vi "Configuration.vi"() -> ()   [LabVIEW 2021]
uses:
  <vilib>/Analysis/Matrix/Datatypes/RealMatrix.ctl
  Sub VIs/Configuration/Configuration.ctl
  <vilib>/Analysis/Matrix/NI_Matrix.lvlib
panel:
  out "values loded in xml files":T1
  in  "file path (trajectorymat)":path=path "c:/ni-rt/startup/new_trajectoryfile.csv"
  in  "file path (matrixmat)":path=path "c:/ni-rt/startup/matrixmat_default.csv"
  in  "Configuration":T2={"Accelerometer Bias"={"X (m/s)"=0.0, "Y (m/s)"=0.5797, "Z (m/s)"=0.0}, "Gyroscope Bias"={"X (m/s)"=0.0, "Y (m/s)"=0.0, "Z (m/s)"=0.0}, "Steering Motor Gear Ratio"=111.0, "Steering Pully Gear Ratio"=1.0, "Steering Encoder CPR"=500.0, "Steering Motor Max RPM"=4000.0, "Wheelbase (m)"=1.12, "Fork Angle (rad)"=1.3, "Balancing Controller"={"Kp (/s)"=1.3, "Kd (1)"=3.0}, "Max Allowed Steering Angle (rad)"=0.7, "Task Periods"={"Emergency Stop (us)"=10000, "IMU (us)"=10000, "Steering Motor Encoder (us)"=10000, "State Estimator (us)"=10000, "Balancing Controller (us)"=10000, "GNSS (us)"=10000, "Logging (us)"=10000, "Drive Motor (us)"=100000, "Visualization (us)"=100000}, "Drive Motor Gear Ratio"=250.0, "lr"=0.4964, "lf"=0.5986, "lambda"=1.2217, "k1"=0.004472, "k2"=0.09678, "e1_max"=11.331, "Ad_tmin"=0.95971, "Bd_tmin"=0.01, "C_tmin"=2.20588, "D_tmin"=0.0, "Wheel radius"=0.311, "Ad_tmax"=0.95971, "Bd_tmax"=0.01, "C_tmax"=2.20588, "D_tmax"=0.0, "Vmin"=2.20588, "Vmax"=0.0}
  in  "Trajectory":dbl[][](array[numeric])=[[5.068129233, 0.5604159844, -0.0872664626], [5.16875496, 0.551612374, -0.0872664626], [5.269380687, 0.5428087636, -0.0872664626], [5.370006414, 0.5340051532, -0.0872664626], [5.470632141, 0.5252015428, -0.0872664626], [5.571257869, 0.5163979325, -0.0872664626], [5.671883596, 0.5075943221, -0.0872664626], [5.772509323, 0.4987907117, -0.0872664626], [5.87313505, 0.4899871013, -0.0872664626], [5.973760777, 0.4811834909, -0.0872664626], [6.074386504, 0.4723798806, -0.0872664626], [6.175012231, 0.4635762702, -0.0872664626], [6.275637958, 0.4547726598, -0.0872664626], [6.376263685, 0.4459690494, -0.0872664626], [6.476889412, 0.4371654391, -0.0872664626], [6.577515139, 0.4283618287, -0.0872664626], [6.678140866, 0.4195582183, -0.0872664626], [6.778766593, 0.4107546079, -0.0872664626], [6.87939232, 0.4019509976, -0.0872664626], [6.980018048, 0.3931473872, -0.0872664626], [7.080643775, 0.3843437768, -0.0872664626], [7.181269502, 0.3755401664, -0.0872664626], [7.281895229, 0.366736556, -0.0872664626], [7.382520956, 0.3579329457, -0.0872664626], [7.483146683, 0.3491293353, -0.0872664626], [7.58377241, 0.3403257249, -0.0872664626], [7.684398137, 0.3315221145, -0.0872664626], [7.785023864, 0.3227185042, -0.0872664626], [7.885649591, 0.3139148938, -0.0872664626], [7.986275318, 0.3051112834, -0.0872664626], [8.086901045, 0.296307673, -0.0872664626], [8.187526772, 0.2875040626, -0.0872664626], [8.288152499, 0.2787004523, -0.0872664626], [8.388778227, 0.2698968419, -0.0872664626], [8.489403954, 0.2610932315, -0.0872664626], [8.590029681, 0.2522896211, -0.0872664626], [8.690655408, 0.2434860108, -0.0872664626], [8.791281135, 0.2346824004, -0.0872664626], [8.891906862, 0.22587879, -0.0872664626], [8.992532589, 0.2170751796, -0.0872664626], [9.093158316, 0.2082715692, -0.0872664626], [9.193784043, 0.1994679589, -0.0872664626], [9.29440977, 0.1906643485, -0.0872664626], [9.395035497, 0.1818607381, -0.0872664626], [9.495661224, 0.1730571277, -0.0872664626], [9.596286951, 0.1642535174, -0.0872664626], [9.696912678, 0.155449907, -0.0872664626], [9.797538405, 0.1466462966, -0.0872664626], [9.898164133, 0.1378426862, -0.0872664626], [9.99878986, 0.1290390758, -0.0872664626], [10.09941559, 0.1202354654, -0.0872664626], [10.20004131, 0.111431855, -0.0872664626], [10.30066704, 0.1026282446, -0.0872664626], [10.40129277, 0.09382463425, -0.0872664626], [10.5019185, 0.08502102387, -0.0872664626], [10.60254422, 0.07621741349, -0.0872664626], [10.70316995, 0.06741380312, -0.0872664626], [10.80379568, 0.05861019274, -0.0872664626], [10.9044214, 0.04980658236, -0.0872664626], [11.00504713, 0.04100297198, -0.0872664626], [11.10567286, 0.03219936161, -0.0872664626], [11.20629859, 0.02339575123, -0.0872664626], [11.30692431, 0.01459214085, -0.0872664626], [11.40755004, 0.005788530473, -0.0872664626], [11.50817577, -0.003015079905, -0.0872664626], [11.60880149, -0.01181869028, -0.0872664626], [11.70942722, -0.02062230066, -0.0872664626], [11.81005295, -0.02942591104, -0.0872664626], [11.91067867, -0.03822952142, -0.0872664626], [12.0113044, -0.04703313179, -0.0872664626], [12.11193013, -0.05583674217, -0.0872664626], [12.21255586, -0.06464035255, -0.0872664626], [12.31318158, -0.07344396293, -0.0872664626], [12.41380731, -0.0822475733, -0.0872664626], [12.51443304, -0.09105118368, -0.0872664626], [12.61505876, -0.09985479406, -0.0872664626], [12.71568449, -0.1086584044, -0.0872664626], [12.81631022, -0.1174620148, -0.0872664626], [12.91693595, -0.1262656252, -0.0872664626], [13.01756167, -0.1350692356, -0.0872664626], [13.1181874, -0.1438728459, -0.0872664626], [13.21881313, -0.1526764563, -0.0872664626], [13.31943885, -0.1614800667, -0.0872664626], [13.42006458, -0.1702836771, -0.0872664626], [13.52069031, -0.1790872875, -0.0872664626], [13.62131604, -0.1878908978, -0.0872664626], [13.72194176, -0.1966945082, -0.0872664626], [13.82256749, -0.2054981186, -0.0872664626], [13.92319322, -0.214301729, -0.0872664626], [14.02381894, -0.2231053393, -0.0872664626], [14.12444467, -0.2319089497, -0.0872664626], [14.2250704, -0.2407125601, -0.0872664626], [14.32569612, -0.2495161705, -0.0872664626], [14.42632185, -0.2583197809, -0.0872664626], [14.52694758, -0.2671233912, -0.0872664626], [14.62757331, -0.2759270016, -0.0872664626], [14.72819903, -0.284730612, -0.0872664626], [14.82882476, -0.2935342224, -0.0872664626], [14.92945049, -0.3023378327, -0.0872664626], [15.03007621, -0.3111414431, -0.0872664626]] format="%#.10g"
  in  "csv matrix":T3=[[1.0, 0.0, 0.0, 0.0, 0.0, 0.0, 0.01], [0.0, 1.0, 0.02, 0.0, 0.0, 0.008519879762, 0.0], [0.0, 0.0, 1.0, 0.0, 0.0, 0.01716333554, 0.0], [0.0, 0.0, 0.0, 1.0, 0.01, 0.0, 0.0], [0.0, 0.0, 0.0, 0.1888354187, 1.0, 0.05678557439, 0.0], [0.0, 0.0, 0.0, 0.0, 0.0, 1.0, 0.0], [0.0, 0.0, 0.0, 0.0, 0.0, 0.0, 1.0], [0.0, 0.0, 0.0, 0.0, 0.01745267886, 0.01, 0.0], [1.0, 0.0, 0.0, 0.0, 0.0, 0.0, 0.0], [0.0, 1.0, 0.0, 0.0, 0.0, 0.0, 0.0], [0.0, 0.0, 0.0, -21.42337825, 0.0, -0.05964571683, 0.0], [0.0, 0.0, 0.0, 0.0, 1.0, 0.0, 0.0], [0.0, 0.0, 0.0, 0.0, 0.0, 1.716333554, 0.0], [0.0, 0.0, 0.0, 0.0, 0.0, 1.0, 0.0], [0.0, 0.0, 0.0, 0.0, 0.0, 0.0, 1.0], [0.0, 0.0, -1.07333975, 0.0, 0.0, 0.0, 0.0], [0.2226851604, 0.0, 0.0, 0.0, 0.0, 0.0, 0.009633547861], [0.0, 0.241922678, 0.0, 0.0, 2.599561845e-05, 0.008475250623, 0.0], [0.0, 0.2205400464, 0.0, 0.0, 5.23683094e-05, 0.01707343673, 0.0], [0.0, 0.0, -6.240552028e-05, 0.01000002817, 0.0, 0.0, 0.0], [0.0, 0.0, -1.233223107e-05, 1.000000005, 0.0001732598335, 0.0564872313, 0.0], [0.0, 0.0, 0.0, 0.0, 0.00305116185, 0.9947584597, 0.0], [6.969070208e-05, 0.0, 0.0, 0.0, 0.0, 0.0, 0.8541018662], [0.0, 0.0, 0.0, 0.0, 0.0, 0.0, 0.0]]
  in  "Stop Program":bool
  in  "Save Configuration":bool
  in  "Load Saved Configuration":bool
  # "e"
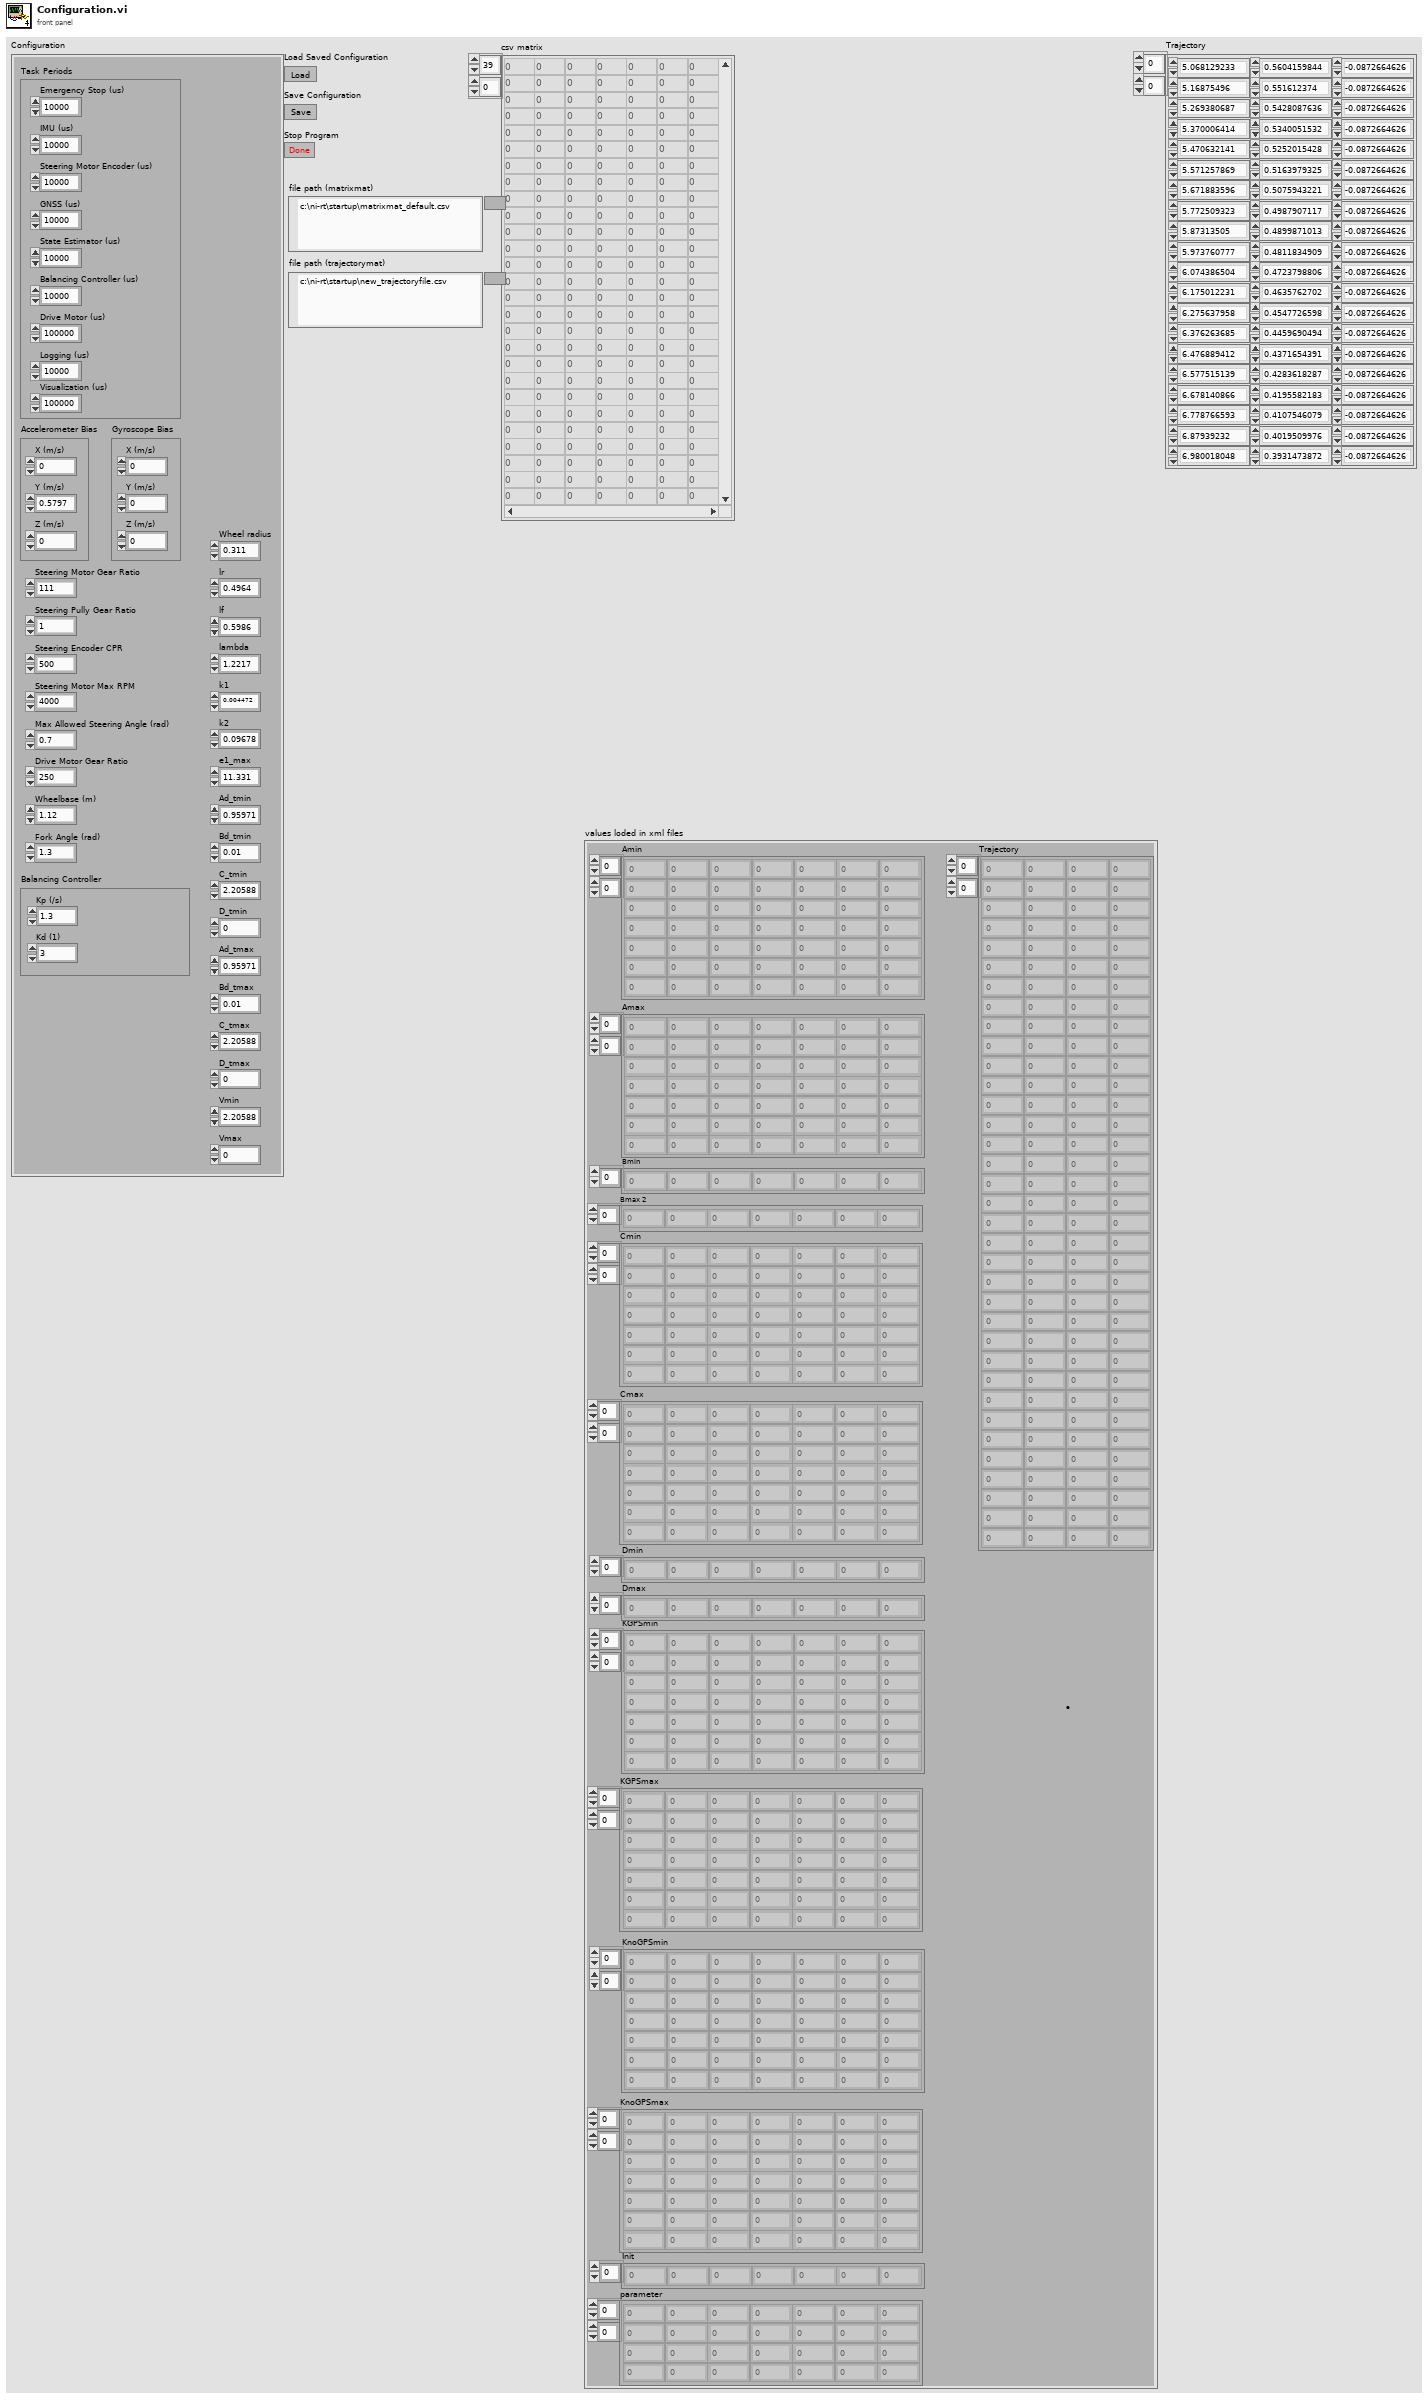
[diagram p1: front panel]
types:
  T1 = cluster{"Bmin":dbl[], "Amin":dbl[][], "Cmin":dbl[][], "Dmin":dbl[], "KGPSmin":dbl[][], "Trajectory":dbl[][], "Init":dbl[], "parameter":dbl[][], "KnoGPSmin":dbl[][], "Amax":dbl[][], "Bmax 2":dbl[], "Cmax":dbl[][], "Dmax":dbl[], "KGPSmax":dbl[][], "KnoGPSmax":dbl[][]}
  T2 = typedef "Configuration.ctl" = cluster{"Accelerometer Bias":cluster{"X (m/s)":dbl, "Y (m/s)":dbl, "Z (m/s)":dbl}, "Gyroscope Bias":cluster{"X (m/s)":dbl, "Y (m/s)":dbl, "Z (m/s)":dbl}, "Steering Motor Gear Ratio":dbl, "Steering Pully Gear Ratio":dbl, "Steering Encoder CPR":dbl, "Steering Motor Max RPM":dbl, "Wheelbase (m)":dbl, "Fork Angle (rad)":dbl, "Balancing Controller":cluster{"Kp (/s)":dbl, "Kd (1)":dbl}, "Max Allowed Steering Angle (rad)":dbl, "Task Periods":cluster{"Emergency Stop (us)":i64, "IMU (us)":i64, "Steering Motor Encoder (us)":i64, "State Estimator (us)":i64, "Balancing Controller (us)":i64, "GNSS (us)":i64, "Logging (us)":i64, "Drive Motor (us)":i64, "Visualization (us)":i64}, "Drive Motor Gear Ratio":dbl, "lr":dbl, "lf":dbl, "lambda":dbl, "k1":dbl, "k2":dbl, "e1_max":dbl, "Ad_tmin":dbl, "Bd_tmin":dbl, "C_tmin":dbl, "D_tmin":dbl, "Wheel radius":dbl, "Ad_tmax":dbl, "Bd_tmax":dbl, "C_tmax":dbl, "D_tmax":dbl, "Vmin":dbl, "Vmax":dbl}
  T3 = typedef "NI_Matrix.lvlib/RealMatrix.ctl" = dbl[][]
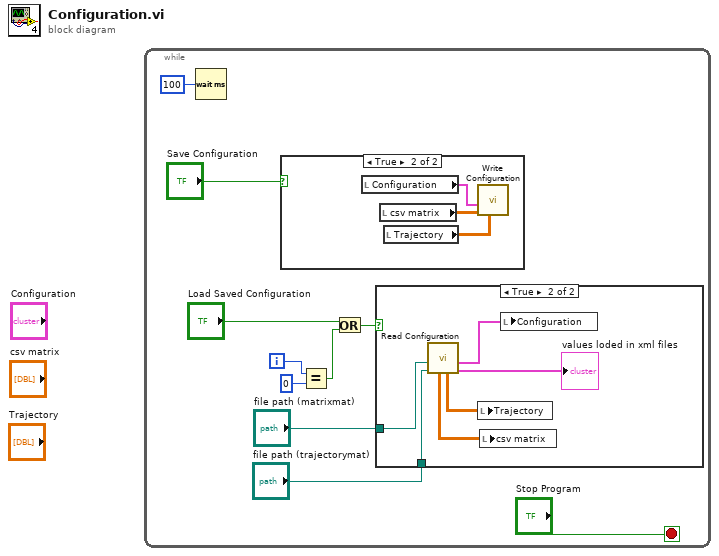
[diagram p0: block diagram]
diagram:
  n1 = while {
    i -> [w7]
    stop <- "Stop Program" stop-if-true
    n2 = Wait (ms)(milliseconds to wait=u32 100) -> ()  [unwired: 1 out]
    n3 = case shown="True" "Save Configuration" {
      frame False {
      }
      frame True {
        n4 = local read "Configuration"() -> (w13:T2)
        n5 = local read "csv matrix"() -> (w12:T3)
        n6 = local read "Trajectory"() -> (w11:dbl[][])
        n7 = call "Write Configuration.vi"("Array"=w11, "Real Matrix"=w12, "Configuration"=w13) -> ()  [unwired: 8 in, 1 out]
      }
    }
    n8 = Equal?(x=w7, y=0) -> (x = y?=w3:bool)
    n9 = Or(x="Load Saved Configuration", y=w3) -> (x .or. y?=w4:bool)
    n10 = case shown="True" w4 {
      tunnel: "file path (matrixmat)" -> [_ w16]
      tunnel: "file path (trajectorymat)" -> [_ w15]
      frame False {
      }
      frame True {
        n11 = call "Read Configuration.vi"("file path (trajectorymat)"=w15, "file path (matrixmat)"=w16) -> ("values loded in xml files"=→"values loded in xml files":T1, "configuration"=w17:T2, "Trajectory"=w19:T3, "Matrix Matlab"=w18:T3)  [unwired: 3 in, 3 out]
        n12 = local write "Trajectory"(w19) -> ()
        n13 = local write "csv matrix"(w18) -> ()
        n14 = local write "Configuration"(w17) -> ()
      }
    }
  }
